vi "Move Stage.vi"(8 "error in (no error)":errorcluster, 9 "Y Axis":dbl, 10 "X Axis":dbl, 11 "2-Axis Stage in":refnum<class "XY Stage Process.lvclass">) -> (0 "error out":errorcluster, 3 "2-Axis Stage out":refnum<class "XY Stage Process.lvclass">)   [LabVIEW 2022 SP3, in "XY Stage Process.lvlib" / "XY Stage Process.lvclass"]
uses:
  XY Stage Process.lvclass
  XY Stage Process.lvclass/XY Stage Process.ctl
  Axis Objects/iMotion Controller/iMotion Controller.lvclass
  Process State Data/Process State Data.lvclass
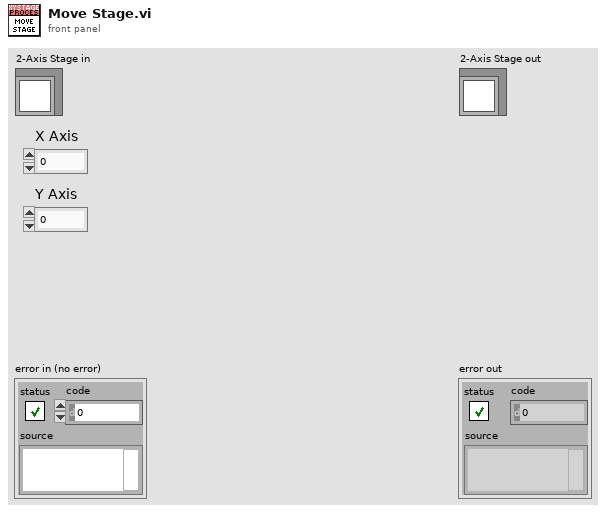
[diagram p1: front panel]
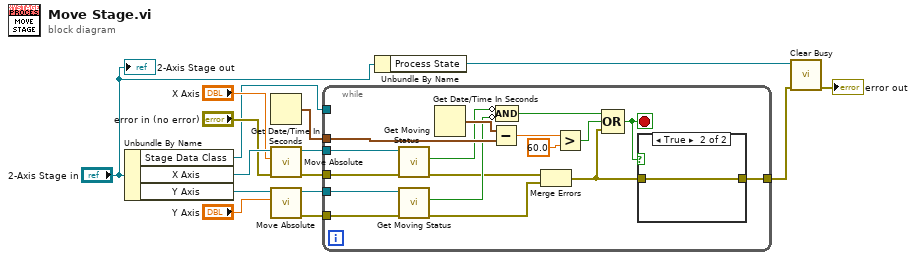
[diagram p0: block diagram]
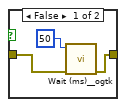
[diagram p2: hidden frame]
diagram:
  n1 = Unbundle By Name("2-Axis Stage in") -> ("Stage Data Class"=w9:refnum<data-value>, "X Axis"=w15:refnum<class "iMotion Controller.lvclass">, "Y Axis"=w14:refnum<class "iMotion Controller.lvclass">)
  n2 = Get Date/Time In Seconds() -> (seconds since 1Jan1904=w10:timestamp)
  n3 = call-dynamic "Move Absolute.vi"("error in (no error)"="error in (no error)", "Desired Position"="X Axis", "iMotion Controller in"=w15) -> ("error out"=w6:errorcluster, "iMotion Controller out"=w8:refnum<class "iMotion Controller.lvclass">)  [unwired: 7 in]
  n4 = call-dynamic "Move Absolute.vi"("Desired Position"="Y Axis", "iMotion Controller in"=w14) -> ("error out"=w5:errorcluster, "iMotion Controller out"=w7:refnum<class "iMotion Controller.lvclass">)  [unwired: 8 in]
  n5 = while {
    tunnel: w6 -> [w19]
    tunnel: [w26] -> w2
    tunnel: w10 -> [w30]
    tunnel: w9 -> [_]
    tunnel: w8 -> [w24]
    tunnel: w7 -> [w23]
    tunnel: w5 -> [w18]
    stop <- w25 stop-if-true
    n6 = call-dynamic "Get Moving Status.vi"("error in (no error)"=w19, "iMotion Controller in"=w24) -> ("error out"=w20:errorcluster, "Moving"=w21:bool)  [unwired: 7 in, 1 out]
    n7 = call-dynamic "Get Moving Status.vi"("error in (no error)"=w18, "iMotion Controller in"=w23) -> ("error out"=w17:errorcluster, "Moving"=w22:bool)  [unwired: 7 in, 1 out]
    n8 = Get Date/Time In Seconds() -> (seconds since 1Jan1904=w31:timestamp)
    n9 = Subtract(x=w31, y=w30) -> (x-y=w28:dbl)
    n10 = Compound Arithmetic op=AND(invert w21, invert w22) -> (w32:bool)
    n11 = Merge Errors(w20, w17) -> (w16:errorcluster)
    n12 = Greater?(x=w28, y=60.0 ("x")) -> (0:w27:bool)
    n13 = Compound Arithmetic op=OR(w32, w27, w16) -> (w25:bool)
    n14 = case shown="True" w25 {
      tunnel: w16 -> [w35 w36]
      tunnel: [w34 w36] -> w26
      frame False {
        n15 = call <userlib>:"Wait (ms)__ogtk.vi"("error in (no error)"=w35, "milliseconds to wait"=u32 50) -> ("error out"=w34:errorcluster)  [unwired: 8 in, 1 out]
      }
      frame True {
      }
    }
  }
  n16 = Unbundle By Name("2-Axis Stage in") -> ("Process State"=w3:refnum<data-value>)
  n17 = call "Clear Busy.vi"("error in (no error)"=w2, "Process State"=w3) -> ("error out"=→"error out":errorcluster)  [unwired: 8 in, 1 out]
  "2-Axis Stage out" <- "2-Axis Stage in"
